vi "dfd_Validate SRate Output Quantizer.vi"(6 "LabVIEW?":bool=TRUE, 8 "error in (no error)":errorcluster, 11 "filter in":T1={"mSRate_Fs"=1.0, "mSRate_Version"="1.0", "mSRate_Comments"="", "mSRate_OrgCoef"={"type"=enum."Undefined", "gain"=1.0, "coef a (k)"=[], "coef b (v)"=[]}, "mSRate_CurCoef"={"type"=enum."Undefined", "gain"=1.0, "coef a (k)"=[], "coef b (v)"=[]}, "mSRate_Quantized?"=FALSE, "mSRate_QCoef"={"type"=enum."Undefined", "gain"=1.0, "coef a (k)"=[], "coef b (v)"=[]}, "mSRate_QSettings"=[], "mSRate_Order"=0, "mSRate_Scaling"={"mSRate_ScaleByPowerOf2?"=FALSE, "mSRate_ScaleType"=enum."No Norm"}} {"mSRate_QSettings"."source" items=["Coef a/k"=0, "Coef b/v"=7, "Input"=1, "Output"=2, "Multiplicand"=3, "Product"=4, "Sum"=5, "Delay"=6, "Gain"=8]}) -> (0 "error out":errorcluster, 3 "filter out":T1={"mSRate_Fs"=1.0, "mSRate_Version"="1.0", "mSRate_Comments"="", "mSRate_OrgCoef"={"type"=enum."Undefined", "gain"=1.0, "coef a (k)"=[], "coef b (v)"=[]}, "mSRate_CurCoef"={"type"=enum."Undefined", "gain"=1.0, "coef a (k)"=[], "coef b (v)"=[]}, "mSRate_Quantized?"=FALSE, "mSRate_QCoef"={"type"=enum."Undefined", "gain"=1.0, "coef a (k)"=[], "coef b (v)"=[]}, "mSRate_QSettings"=[], "mSRate_Order"=0, "mSRate_Scaling"={"mSRate_ScaleByPowerOf2?"=FALSE, "mSRate_ScaleType"=enum."No Norm"}} {"mSRate_QSettings"."source" items=["Coef a/k"=0, "Coef b/v"=7, "Input"=1, "Output"=2, "Multiplicand"=3, "Product"=4, "Sum"=5, "Delay"=6, "Gain"=8]})   [LabVIEW 2017, in "NI_DigFilterLicensed.lvlib"]
uses:
  <vilib>/addons/Digital Filter Design/NI_DigFilterLicensed.lvlib
  <vilib>/addons/Digital Filter Design/_Objects.llb/DFD Filter Obj.ctl
  <vilib>/addons/Digital Filter Design/_Objects.llb/DFD Filter Coef.ctl
  <vilib>/addons/Digital Filter Design/_Objects.llb/DFD Filter Structure Type Selector.ctl
  <vilib>/addons/Digital Filter Design/_Objects.llb/dfd_Internal Quantization Settings.ctl
  <vilib>/addons/Digital Filter Design/_Objects.llb/dfd_Internal Quantization Srcs.ctl
  <vilib>/addons/Digital Filter Design/_Objects.llb/DFD Coef Norm Type.ctl
  <vilib>/addons/Digital Filter Design/_Misc.llb/dfd_Error Handlers (Multiple).vi
  <vilib>/addons/Digital Filter Design/NI_DigFilter_FXP.lvlib
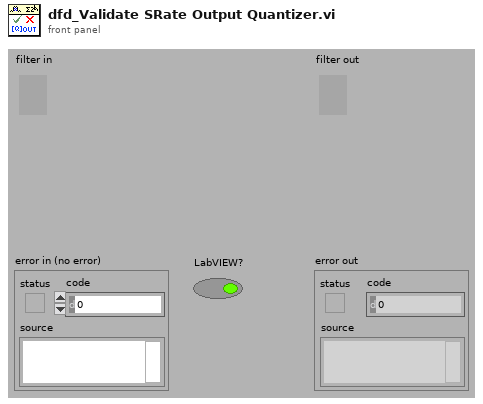
[diagram p1: front panel]
types:
  T1 = typedef "NI_DigFilterLicensed.lvlib/DFD Filter Obj.ctl" = cluster{"mSRate_Fs":dbl, "mSRate_Version":string, "mSRate_Comments":string, "mSRate_OrgCoef":T2, "mSRate_CurCoef":T2, "mSRate_Quantized?":bool, "mSRate_QCoef":T2, "mSRate_QSettings":T4[], "mSRate_Order":i32, "mSRate_Scaling":cluster{"mSRate_ScaleByPowerOf2?":bool, "mSRate_ScaleType":T6}}
  T2 = typedef "NI_DigFilterLicensed.lvlib/DFD Filter Coef.ctl" = cluster{"type":T3, "gain":dbl, "coef a (k)":dbl[], "coef b (v)":dbl[]}
  T3 = typedef "NI_DigFilterLicensed.lvlib/DFD Filter Structure Type Selector.ctl" = enum16{"Undefined", "FIR Direct Form", "FIR Direct Form Transposed", "FIR Symmetric", "FIR Antisymmetric", "IIR Direct Form I", "IIR Direct Form I Transposed", "IIR Direct Form II", "IIR Direct Form II Transposed", "IIR Cascaded Second Order Sections Form I", "IIR Cascaded Second Order Sections Form I Transposed", "IIR Cascaded Second Order Sections Form II", "IIR Cascaded Second Order Sections Form II Transposed", "Lattice Allpass (basic sections)", "Lattice Allpass (one multiplier sections)", "Lattice Allpass (normalized sections)", "Lattice AR (basic sections)", "Lattice AR (one multiplier sections)", "Lattice AR (normalized sections)", "Lattice MA (minimum phase)", "Lattice MA (maximum phase)", "Lattice ARMA (basic sections)", "Lattice ARMA (one multiplier sections)", "Lattice ARMA (normalized sections)"}
  T4 = typedef "NI_DigFilterLicensed.lvlib/dfd_Internal Quantization Settings.ctl" = cluster{"source":T5, "wl":i16, "iwl":i16, "overflow mode":enum16{"Saturation", "Wrap"}, "rounding mode":enum16{"Nearest", "Truncation"}, "signed?":bool}
  T5 = typedef "NI_DigFilterLicensed.lvlib/dfd_Internal Quantization Srcs.ctl" = u16
  T6 = typedef "NI_DigFilterLicensed.lvlib/DFD Coef Norm Type.ctl" = enum16{"No Norm", "Time Domain 1-Norm", "Time Domain 2-Norm", "Time Domain Inf-Norm"}
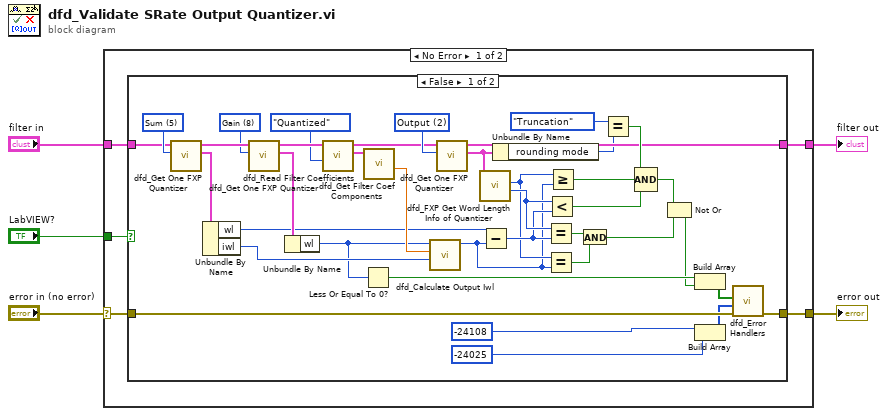
[diagram p0: block diagram]
diagram:
  n1 = case shown="No Error" "error in (no error)" {
    selector: "error in (no error)" -> [w9 w52]
    tunnel: "LabVIEW?" -> [w10 _]
    tunnel: [w8 w52] -> w3
    tunnel: "filter in" -> [w7 w51]
    tunnel: [w6 w51] -> w1
    frame No Error {
      n2 = case shown="False" w10 {
        tunnel: w9 -> [w21 w50]
        tunnel: [w20 w50] -> w8
        tunnel: w7 -> [w47 w49]
        tunnel: [w19 w49] -> w6
        frame False {
          w37 = T5 2 items=["Coef a/k"=0, "Coef b/v"=7, "Input"=1, "Output"=2, "Multiplicand"=3, "Product"=4, "Sum"=5, "Delay"=6, "Gain"=8] ("quantization source")
          w45 = T5 8 items=["Coef a/k"=0, "Coef b/v"=7, "Input"=1, "Output"=2, "Multiplicand"=3, "Product"=4, "Sum"=5, "Delay"=6, "Gain"=8] ("quantization source")
          w48 = T5 5 items=["Coef a/k"=0, "Coef b/v"=7, "Input"=1, "Output"=2, "Multiplicand"=3, "Product"=4, "Sum"=5, "Delay"=6, "Gain"=8] ("quantization source")
          n3 = call <vilib>:"dfd_Get One FXP Quantizer.vi"("quantization source"=w48, "filter in"=w47) -> ("quantization settings"=w44:T4, "filter out"=w46:T1)  [unwired: 1 in, 7 out]
          n4 = Unbundle By Name(w44) -> ("wl"=w34:i16, "iwl"=w39:i16)
          n5 = call <vilib>:"dfd_Get One FXP Quantizer.vi"("quantization source"=w45, "filter in"=w46) -> ("quantization settings"=w40:T4, "filter out"=w43:T1)  [unwired: 1 in, 7 out]
          n6 = Unbundle By Name(w40) -> ("wl"=w17:i16)
          n7 = call <vilib>:"dfd_Read Filter Coefficients.vi"("coef source"=enum16{"Original", "Current", "Quantized"}."Quantized", "filter in"=w43) -> ("filter coef"=w41:T2, "filter out"=w36:T1)  [unwired: 1 in, 7 out]
          n8 = Less Or Equal To 0?(x=w17) -> (x <= 0?=w16:bool)
          n9 = call <vilib>:"dfd_Get Filter Coef Components.vi"("filter coef"=w41) -> ("gain"=w38:dbl)  [unwired: 1 in, 9 out]
          n10 = call <vilib>:"dfd_Calculate Output Iwl.vi"("sum iwl"=w39, "gain value"=w38, "gain wl"=w17) -> ("output iwl"=w28:i16)  [unwired: 8 out]
          n11 = call <vilib>:"dfd_Get One FXP Quantizer.vi"("quantization source"=w37, "filter in"=w36) -> ("quantization settings"=w35:T4, "filter out"=w19:T1)  [unwired: 1 in, 7 out]
          n12 = call <vilib>:"dfd_FXP Get Word Length Info of Quantizer.vi"("quantization settings"=w35) -> ("fwl"=w31:i16, "iwl"=w29:i16)  [unwired: 9 out]
          n13 = Subtract(x=w34, y=w28) -> (x-y=w30:i16)
          n14 = Unbundle By Name(w35) -> ("rounding mode"=w18:enum16{"Nearest", "Truncation"})
          n15 = Equal?(x=w31, y=w30) -> (x = y?=w33:bool)
          n16 = Equal?(x=w29, y=w28) -> (x = y?=w32:bool)
          n17 = Less?(x=w31, y=w30) -> (x < y?=w24:bool)
          n18 = Greater Or Equal?(x=w29, y=w28) -> (x >= y?=w25:bool)
          n19 = And(x=w33, y=w32) -> (x .and. y?=w22:bool)
          n20 = Equal?(x=enum16{"Nearest", "Truncation"}."Truncation", y=w18) -> (x = y?=w26:bool)
          n21 = Compound Arithmetic op=AND(w26, w25, w24) -> (w23:bool)
          n22 = Not Or(1:w22, 2:w23) -> (0:w15:bool)
          n23 = Build Array(w16, w15) -> (w14:bool[])
          n24 = Build Array(-24108 ("ERR_C_CODEGEN_GAIN_ONTARGET"), -24025 ("ERR_CODE_UNSUPPORT_MODEL")) -> (w11:i32[])
          n25 = call-poly <vilib>:"dfd_Error Handlers.vi"("error in (no error)"=w21, "error sources"=w11, "condition failed?"=w14) -> ("error out"=w20:errorcluster)  [unwired: 8 out]
        }
        frame True {
        }
      }
    }
    frame Error {
    }
  }
  "filter out" <- w1
  "error out" <- w3
